vi "Reinitialize.vi"(8 "error in (no error)":errorcluster, 11 "MKS MF1 in":refnum<class "PL MKS MF1 USB.lvclass">) -> (0 "error out":errorcluster, 3 "MKS MF1 out":refnum<class "PL MKS MF1 USB.lvclass">)   [LabVIEW 2015, in "PL MKS MF1 USB.lvclass"]
doc: "Reinitializes connection to device based on previously specified settings."
uses:
  PL MKS MF1 USB.lvclass
  PL MKS MF1 USB.lvclass/PL MKS MF1 USB.ctl
  <vilib>/Instr/_visa.llb/VISA Configure Serial Port (Instr).vi
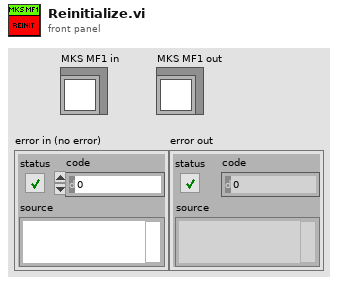
[diagram p1: front panel]
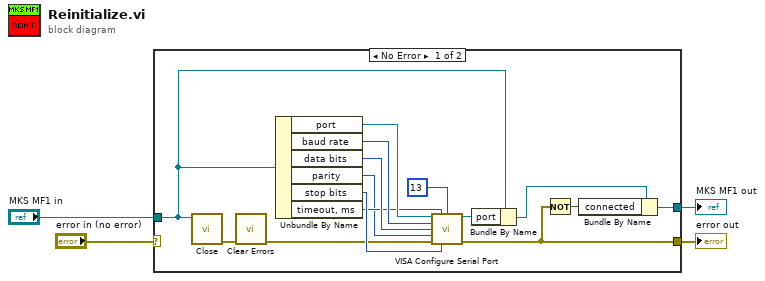
[diagram p0: block diagram]
diagram:
  n1 = case shown="No Error" "error in (no error)" {
    selector: "error in (no error)" -> [_ w20]
    tunnel: "MKS MF1 in" -> [w19 w21]
    tunnel: [w16 w21] -> w3
    tunnel: [w7 w20] -> w2
    frame No Error {
      n2 = call "Close.vi"("MKS MF1 in"=w19) -> ("error out"=w10:errorcluster)  [unwired: 10 in]
      n3 = call <vilib>:"Clear Errors.vi"("error in (no error)"=w10) -> ("error out"=w9:errorcluster)  [unwired: 5 in, 1 out]
      n4 = Unbundle By Name(w19) -> ("port"=w12:refnum<visa-resource-name>, "baud rate"=w15:u32, "data bits"=w14:u16, "parity"=w6:enum16{"None", "Odd", "Even", "Mark", "Space"}, "stop bits"=w13:u16, "timeout, ms"=w11:u32)
      n5 = call-poly "VISA Configure Serial Port"("VISA resource name"=w12, "timeout (10sec)"=w11, "termination char\n(0xA = '\\n' = LF)"=u8 13 ("termination char\n(0xA = '\\n' = LF)"), "baud rate (9600)"=w15, "data bits (8)"=w14, "parity (0:none)"=w6, "error in (no error)"=w9, "stop bits (10: 1 bit)"=w13) -> ("VISA resource name out"=w8:refnum<visa-resource-name>, "error out"=w7:errorcluster)  [unwired: 6 in]
      n6 = Bundle By Name(cluster=w19, "port"=w8) -> (w18:refnum<class "PL MKS MF1 USB.lvclass">)
      n7 = Not(x=w7) -> (.not. x?=w17:bool)
      n8 = Bundle By Name(cluster=w18, "connected"=w17) -> (w16:refnum<class "PL MKS MF1 USB.lvclass">)
    }
    frame Error {
    }
  }
  "MKS MF1 out" <- w3
  "error out" <- w2
